vi "Finish.vi"   [LabVIEW 2013]
doc: "This VI is called just before exiting. It is expected to close I/O refnum, save collected data, etc."
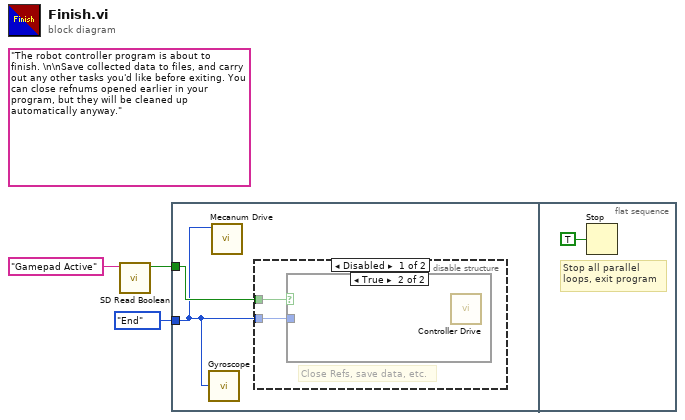
[diagram p0: block diagram]
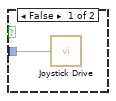
[diagram p2: hidden frame]
diagram:
  (unwired) "The robot controller program is about to finish. \n\nSave collected data to files, and carry out any other tasks you'd like before exiting. You can close refnums opened earlier in your program, but they will be cleaned up automatically anyway."
  n1 = call <vilib>:"SD Read Boolean.vi"("Name"="Gamepad Active") -> ("Boolean"=w1:bool)  [unwired: 8 in, 2 out]
  n2 = flat-sequence {
    tunnel: enum16{"Open", "Run", "End"}."End" ("State Control") -> [w4]
    tunnel: w1 -> [w5]
    frame #0 {
      n3 = call "Gyroscope.vi"("State Control"=w4) -> ()  [unwired: 1 in]
      n4 = call "Mecanum Drive.vi"("State Control"=w4) -> ()  [unwired: 3 in]
      n5 = disable-structure shown="Disabled" {
        disable-tunnel: w5 -> [w7 _]
        disable-tunnel: w4 -> [w6 _]
        frame Disabled {
          # "Close Refs, save data, etc."
          n6 = case shown="True" w7 {
            tunnel: w6 -> [w8 _]
            frame False {
              n7 = call "Joystick Drive.vi"("State"=w8) -> ()
            }
            frame True {
              n8 = call "Controller Drive.vi"() -> ()  [unwired: 1 in]
            }
          }
        }
        frame Enabled {
        }
      }
    }
    frame #1 {
      # "Stop all parallel\nloops, exit program"
      n9 = Stop(stop? (T)=TRUE ("Quit")) -> ()
    }
  }
